vi "Brain.vi"() -> ()   [LabVIEW 2017]
uses:
  <vilib>/OPCUA/controls/NodeId.ctl
  <vilib>/OPCUA/controls/Write Status.ctl
  <vilib>/Utility/file.llb/Read Delimited Spreadsheet (string).vi
  <vilib>/Utility/file.llb/Write Delimited Spreadsheet (string).vi
  <vilib>/OPCUA/client/Multiple Write Double Array.vi
  <vilib>/Utility/file.llb/Write Delimited Spreadsheet (DBL).vi
  <resource>/objmgr/ni.dex.rc
  <vilib>/OPCUA/NI OPC UA Client.lvlib
panel:
  in  "VFD Stop":bool
  in  "Shutdown":bool
  out "Remote VI Error Messages":string
  in  "Node Status":u32
  in  "Time Stamp":timestamp
  in  "Error In":errorcluster
  out "Error Out":errorcluster
  in  "Stop DAQ":bool
  out "DAQ?":bool
  out "Available Elements for Reading":i32
  out "Number of Disconnections":u32
  out "System Loop Time (ms)":u32
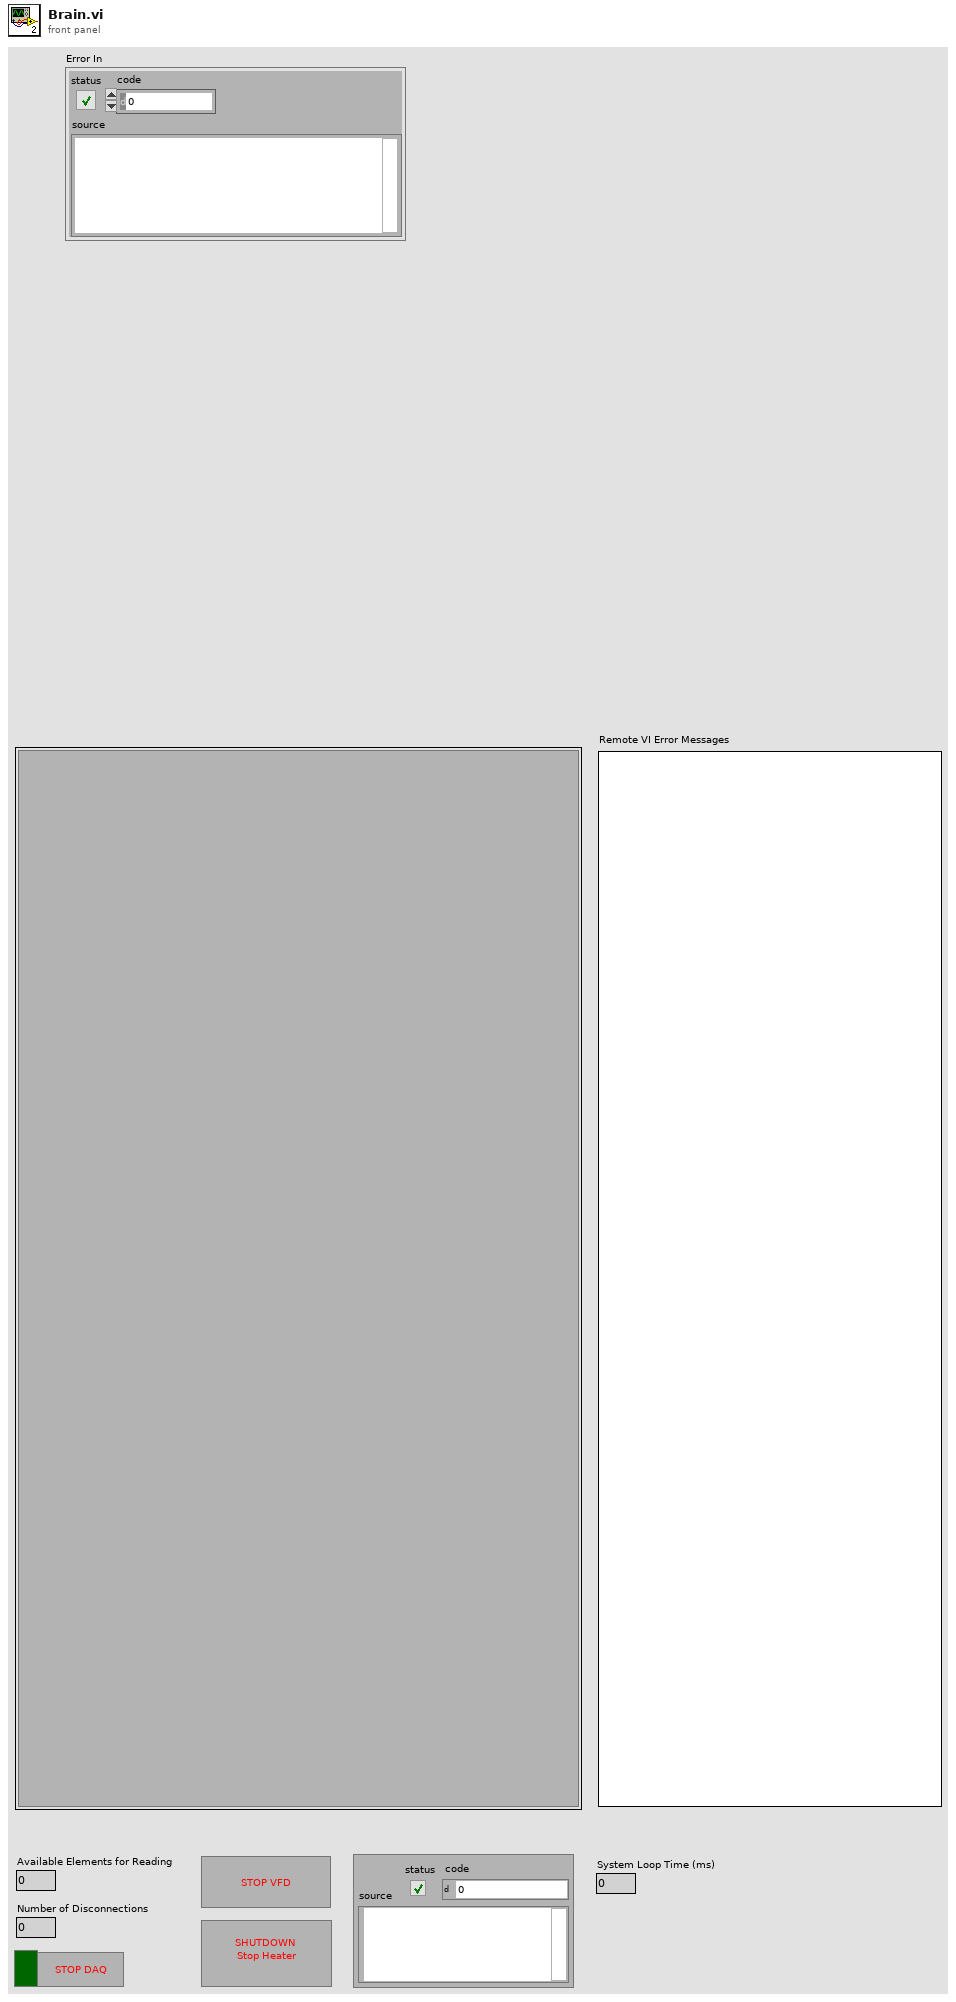
[diagram p1: front panel]
types:
  T1 = typedef "OPC UA Client Refnum.ctl" = refnum<k21>
  T2 = typedef "NodeId.ctl" = string
  T3 = typedef "Write Status.ctl" = u32
  T4 = cluster{"node ID":T2, "value":dbl[], "timestamp (current time)":timestamp, "node status":T3}
  T5 = cluster{"node ID":T2, "value":dbl[], "timestamp (current time)":timestamp, "node status":T3}[]
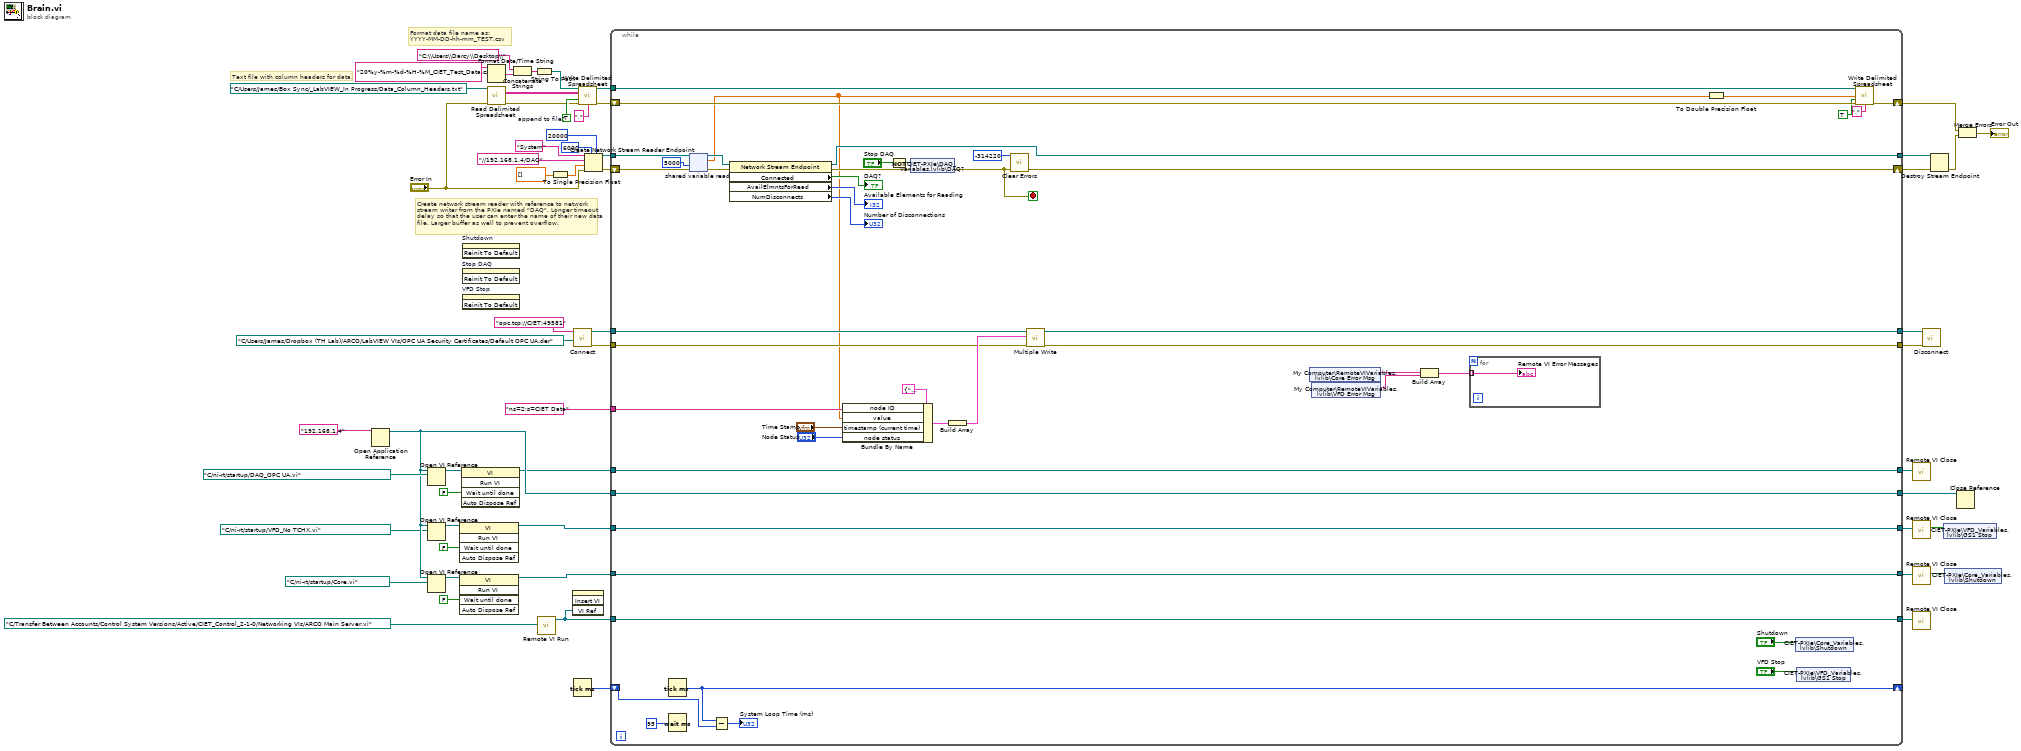
[diagram p0: block diagram]
diagram:
  w44 = TRUE  # append to file?
  # "Format data file name as:\nYYYY-MM-DD-hh-mm_TEST.csv"
  # "Create network stream reader with reference to network\nstream writer from the PXIe named \"DAQ\". Longer timeout\ndelay so that the user can enter the name of their new data\nfile. Larger buffer as well to prevent overflow."
  # "Text file with column headers for data."
  n1 = Open Application Reference(11:"192.168.1.4" ("machine name (\"\":  open local reference)")) -> (3:w14:refnum<vi>)  [unwired: 3 in, 1 out]
  n2 = Open VI Reference(application reference (local)=w14, vi path=path "C:/ni-rt/startup/DAQ_OPC UA.vi") -> (vi reference=w11:refnum<vi>)  [unwired: 4 in, 1 out]
  n3 = Open VI Reference(application reference (local)=w14, vi path=path "C:/ni-rt/startup/VFD_No TCHX.vi") -> (vi reference=w9:refnum<vi>)  [unwired: 4 in, 1 out]
  n4 = Open VI Reference(application reference (local)=w14, vi path=path "C:/ni-rt/startup/Core.vi") -> (vi reference=w7:refnum<vi>)  [unwired: 4 in, 1 out]
  n5 = invoke class="VI" method="Run VI"(reference=w9, "Wait until done"=FALSE ("Wait Until Done")) -> (reference out=w8:refnum<vi>)  [unwired: 3 in, 4 out]
  n6 = invoke class="VI" method="Run VI"(reference=w7, "Wait until done"=FALSE ("Wait Until Done")) -> (reference out=w6:refnum<vi>)  [unwired: 3 in, 4 out]
  n7 = invoke class="VI" method="Run VI"(reference=w11, "Wait until done"=FALSE ("Wait Until Done")) -> (reference out=w10:refnum<vi>)  [unwired: 3 in, 4 out]
  n8 = invoke on="Shutdown" class="Bool (strict)" method="Reinit To Default"() -> ()  [unwired: 3 in, 3 out]
  n9 = invoke on="Stop DAQ" class="Bool (strict)" method="Reinit To Default"() -> ()  [unwired: 3 in, 3 out]
  n10 = invoke on="VFD Stop" class="Bool (strict)" method="Reinit To Default"() -> ()  [unwired: 3 in, 3 out]
  n11 = Format Date/Time String(time format string (%c)="20%y-%m-%d-%H-%M_CIET_Test_Data.csv") -> (date/time string=w34:string)  [unwired: 2 in]
  n12 = call-poly <vilib>:"Read Delimited Spreadsheet.vi"("file path (dialog if empty)"=path "C:/Users/James/Box Sync/_LabVIEW_In Progress/Data_Column_Headers.txt", "error in (no error)"="Error In") -> ("all rows"=w47:string[][], "error out"=w42:errorcluster)  [unwired: 8 in, 4 out]
  n13 = Concatenate Strings("C:\\Users\\Darcy\\Desktop\\" ("string"), w34) -> (w36:string)
  n14 = String To Path(string=w36) -> (path=w33:path)
  n15 = call "Remote VI Run.vi"("VI Path"=path "C:/Transfer Between Accounts/Control System Versions/Active/CIET_Control_2-1-0/Networking VIs/ARCO Main Server.vi" ("vi path")) -> ("VI Reference"=w17:refnum<vi>)  [unwired: 10 in]
  n16 = To Single Precision Float(number=dbl[] []) -> (single precision float=w55:sgl[])
  n17 = invoke on="Sub Panel" class="SubPnl" method="Insert VI"("VI Ref"=w17) -> ()  [unwired: 3 in, 4 out]
  n18 = call <vilib>:"Connect.vi"("client certificate file"=path "C:/Users/James/Dropbox (TH Lab)/ARCO/LabVIEW VIs/OPC UA Security Certificates/Default OPC UA.der", "server endpoint URL"="opc.tcp://CIET:49581") -> ("error out"=w27:errorcluster, "OPC UA client refnum out"=w28:T1)  [unwired: 7 in, 1 out]
  n19 = Tick Count (ms)() -> (millisecond timer value=w31:u32)
  n20 = call-poly <vilib>:"Write Delimited Spreadsheet.vi"("file path (dialog if empty)"=w33, "2D data"=w47, "append to file? (new file:F)"=w44, "error in (no error)"=w42, "delimiter (\\t)"=",") -> ("new file path (Not A Path if cancelled)"=w43:path, "error out"=w41:errorcluster)  [unwired: 9 in]
  n21 = Create Network Stream Reader Endpoint(5:20000 ("timeout in ms (-1)"), 7:6000 ("reader buffer size"), 8:"Error In", 9:w55, 10:"//192.168.1.4/DAQ" ("writer url"), 11:"System" ("reader name")) -> (0:w52:errorcluster, 3:w51:refnum<k21>)  [unwired: 1 in]
  n22 = while {
    shift-right: [w92] -> w50
    shift-left: w52 -> [w100]
    tunnel: w51 -> [w101]
    tunnel: [w91] -> w49
    tunnel: w43 -> [w87]
    shift-right: [w85] -> w40
    shift-left: w41 -> [w86]
    shift-right: [w80] -> _
    shift-left: w31 -> [w81]
    tunnel: w28 -> [w73]
    tunnel: w27 -> [w72]
    tunnel: "ns=2;s=CIET Data" -> [w71]
    tunnel: [w69] -> w25
    tunnel: [w68] -> w24
    tunnel: w10 -> [w67]
    tunnel: [w67] -> w22
    tunnel: w14 -> [w66]
    tunnel: [w66] -> w21
    tunnel: w8 -> [w65]
    tunnel: [w65] -> w20
    tunnel: w6 -> [w64]
    tunnel: [w64] -> w19
    tunnel: w17 -> [w63]
    tunnel: [w63] -> w18
    stop <- w90 stop-if-true
    n23 = Tick Count (ms)() -> (millisecond timer value=w80:u32)
    n24 = Wait (ms)(milliseconds to wait=u32 95) -> ()  [unwired: 1 out]
    n25 = shared-variable-read(w101, w100, 5000 ("timeout ms (-1)")) -> (w97:refnum<k21>, w95:errorcluster, w70:sgl[])  [unwired: 1 out]
    n26 = Subtract(x=w80, y=w81) -> (x-y=→"System Loop Time (ms)":u32)
    n27 = property class="Network Stream Endpoint"(reference=w97, error in=w95) -> (reference out=w91:refnum<k21>, error out=w96:errorcluster, "Connected"=→"DAQ?":bool, "AvailElmntsForRead"=→"Available Elements for Reading":i32, "NumDisconnects"=→"Number of Disconnections":u32)
    n28 = Bundle By Name(cluster=T4 {"node ID"="", "value"=[], "timestamp (current time)"=timestamp(0 s since 1904-01-01), "node status"=0} ("request"), "node ID"=w71, "value"=w70, "timestamp (current time)"="Time Stamp", "node status"="Node Status") -> (w75:T4)
    n29 = Not(x="Stop DAQ") -> (.not. x?=w99:bool)
    n30 = shared-variable "CIET-PXIe\\DAQ_Variables.lvlib\\DAQ?"(w99, error in=w96) -> (error out=w90:errorcluster)
    n31 = Build Array(w75) -> (w74:T5)
    n32 = call <vilib>:"Clear Errors.vi"("error in (no error)"=w90, "specific error code to clear (0: all)"=-314220) -> ("error out"=w92:errorcluster)  [unwired: 4 in, 1 out]
    n33 = call-poly <vilib>:"Multiple Write.vi"("error in (no error)"=w72, "requests"=w74, "OPC UA client refnum in"=w73) -> ("error out"=w68:errorcluster, "OPC UA client refnum out"=w69:T1)  [unwired: 5 in, 2 out]
    n34 = shared-variable "My Computer\\RemoteVIVariables.lvlib\\Core Error Msg"() -> (w62:string)  [unwired: 1 in, 1 out]
    n35 = shared-variable "My Computer\\RemoteVIVariables.lvlib\\VFD Error Msg"() -> (w61:string)  [unwired: 1 in, 1 out]
    n36 = Build Array(w62, w61) -> (w60:string[])
    n37 = for {
      tunnel: w60 -> [w104] mode=indexing
      "Remote VI Error Messages" <- w104
    }
    n38 = To Double Precision Float(number=w70) -> (double precision float=w82:dbl[])
    n39 = shared-variable "CIET-PXIe\\Core_Variables.lvlib\\Shutdown"("Shutdown") -> ()  [unwired: 1 in, 1 out]
    n40 = shared-variable "CIET-PXIe\\VFD_Variables.lvlib\\GS1 Stop"("VFD Stop") -> ()  [unwired: 1 in, 1 out]
    n41 = call-poly <vilib>:"Write Delimited Spreadsheet.vi"("file path (dialog if empty)"=w87, "1D data"=w82, "append to file? (new file:F)"=TRUE, "error in (no error)"=w86, "delimiter (\\t)"="," ("delimiter (\\t)")) -> ("error out"=w85:errorcluster)  [unwired: 9 in, 1 out]
  }
  n42 = call "Remote VI Close.vi"("reference"=w22) -> ()  [unwired: 10 in, 1 out]
  n43 = call "Remote VI Close.vi"("reference"=w20) -> ("SubVI Stop"=w1:bool)  [unwired: 10 in]
  n44 = call "Remote VI Close.vi"("reference"=w19) -> ("SubVI Stop"=w2:bool)  [unwired: 10 in]
  n45 = call "Remote VI Close.vi"("reference"=w18) -> ()  [unwired: 10 in, 1 out]
  n46 = call <vilib>:"Disconnect.vi"("error in (no error)"=w24, "OPC UA client refnum in"=w25) -> ()  [unwired: 9 in, 1 out]
  n47 = Destroy Stream Endpoint(8:w50, 11:w49) -> (0:w39:errorcluster)
  n48 = shared-variable "CIET-PXIe\\VFD_Variables.lvlib\\GS1 Stop"(w1) -> ()  [unwired: 1 in, 1 out]
  n49 = shared-variable "CIET-PXIe\\Core_Variables.lvlib\\Shutdown"(w2) -> ()  [unwired: 1 in, 1 out]
  n50 = Close Reference(reference=w21) -> ()  [unwired: 1 in, 1 out]
  n51 = Merge Errors(w40, w39) -> (→"Error Out":errorcluster)
